vi "BM_add.vi"(7 "LabVIEW Web Service Request":refnum<class "Web Request.lvclass"> caption="LabVIEW Web服务请求", 8 "fenhang":string, 9 "name":string, 10 "id":string, 11 "action":string) -> (0 "error":errorcluster, 6 "data2":string[][](array[string]) caption="查询数据")   [LabVIEW 2017]
uses:
  <vilib>/wsapi/Web Request.lvclass
panel:
  out "postdata":string caption="post数据"
  out "error out":errorcluster caption="错误输出"
  # "Web服务请求输入接线端用于调用“Web服务”选板的VI。除非不需要访问该选板，否则不要在连线板上删除这个输入接线端。"
  # "添加至连线板的每一个其他输入控件，在URL中对应于一个输入。如需在接线端模式输出（默认设置）下包含显示控件，则该显示控件必须与连线板相连。"
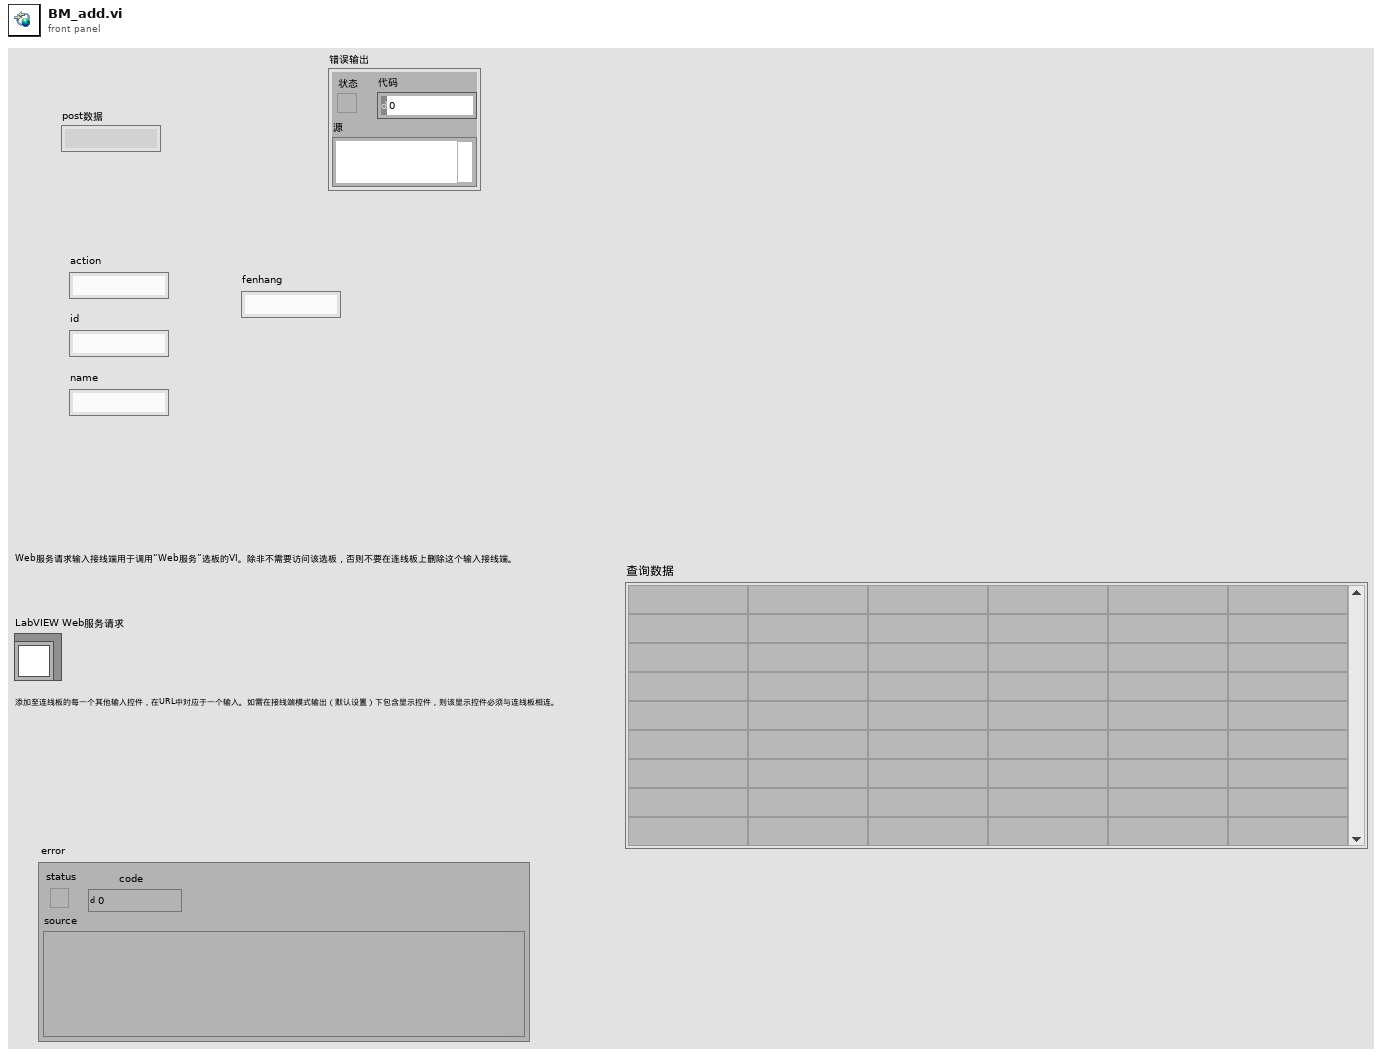
[diagram p1: front panel]
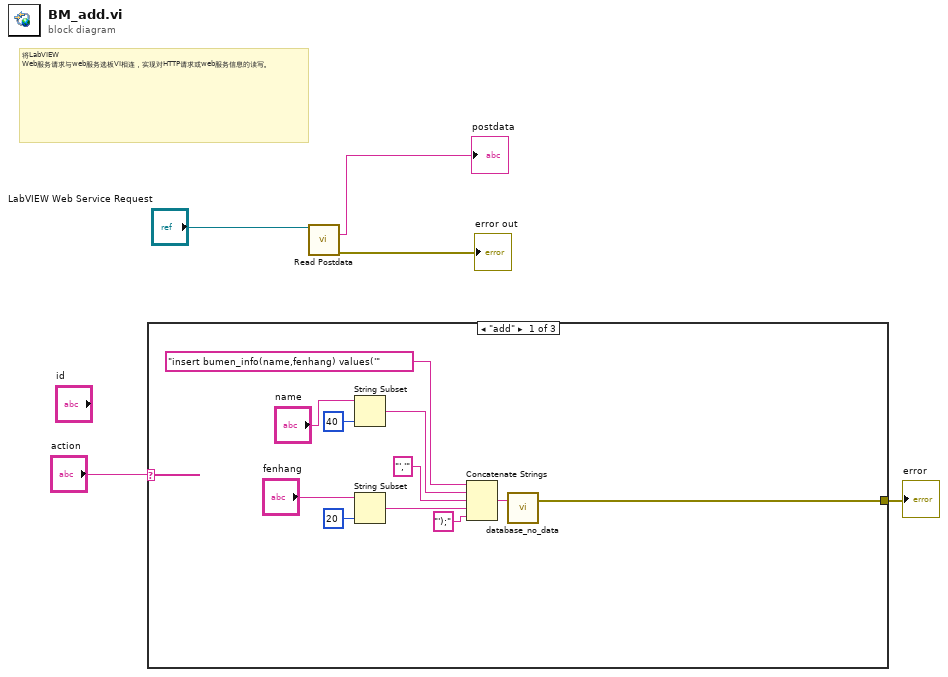
[diagram p0: block diagram]
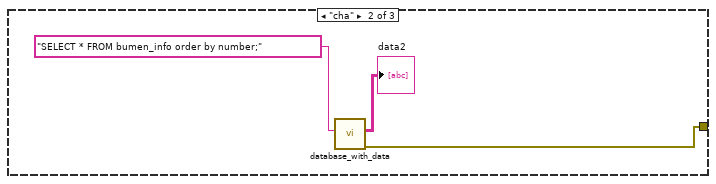
[diagram p2: hidden frame]
diagram:
  # "将LabVIEW Web服务请求与web服务选板VI相连，实现对HTTP请求或web服务信息的读写。"
  n1 = case shown="\"add\"" "action" {
    tunnel: [w6 w17 _] -> w1
    frame "add" {
      n2 = String Subset(string="name", length (rest)=40 ("长度（剩余）")) -> (substring=w14:string)  [unwired: 1 in]
      n3 = String Subset(string="fenhang", length (rest)=20 ("长度（剩余）")) -> (substring=w8:string)  [unwired: 1 in]
      n4 = Concatenate Strings("insert bumen_info(name,fenhang) values('" ("格式字符串"), w14, "','" ("字符串"), w8, "');" ("字符串")) -> (w7:string)
      n5 = call "database_no_data.vi"("input"=w7) -> ("error"=w6:errorcluster)  [unwired: 2 in]
    }
    frame "cha" {
      n6 = call "database_with_data.vi"("input"="SELECT * FROM bumen_info order by number;" ("格式字符串")) -> ("error"=w17:errorcluster, "Data"=→"data2":string[][])  [unwired: 9 in]
    }
    frame Default {
    }
  }
  "error" <- w1
  n7 = call <vilib>:"Read Postdata.vi"("LabVIEW Web Service Request"="LabVIEW Web Service Request") -> ("postdata"=→"postdata":string, "error out"=→"error out":errorcluster)  [unwired: 12 in, 1 out]
